vi "infoStepMini.vi"(8 "error in (no error)":errorcluster, 10 "StepId":i32, 11 "Array":T1[](array[typedef])) -> (0 "error out":errorcluster, 3 "Info Test":string)   [LabVIEW 2019]
doc: "Riassume le informazioni principali degli step in un formato più leggibile e ridotto"
uses:
  ByteQXAPIBase/TypeDef/Step.ctl
  ByteQXAPIBase/TypeDef/Asset.ctl
  ByteQXAPIBase/ByteQXAPIBase.lvclass
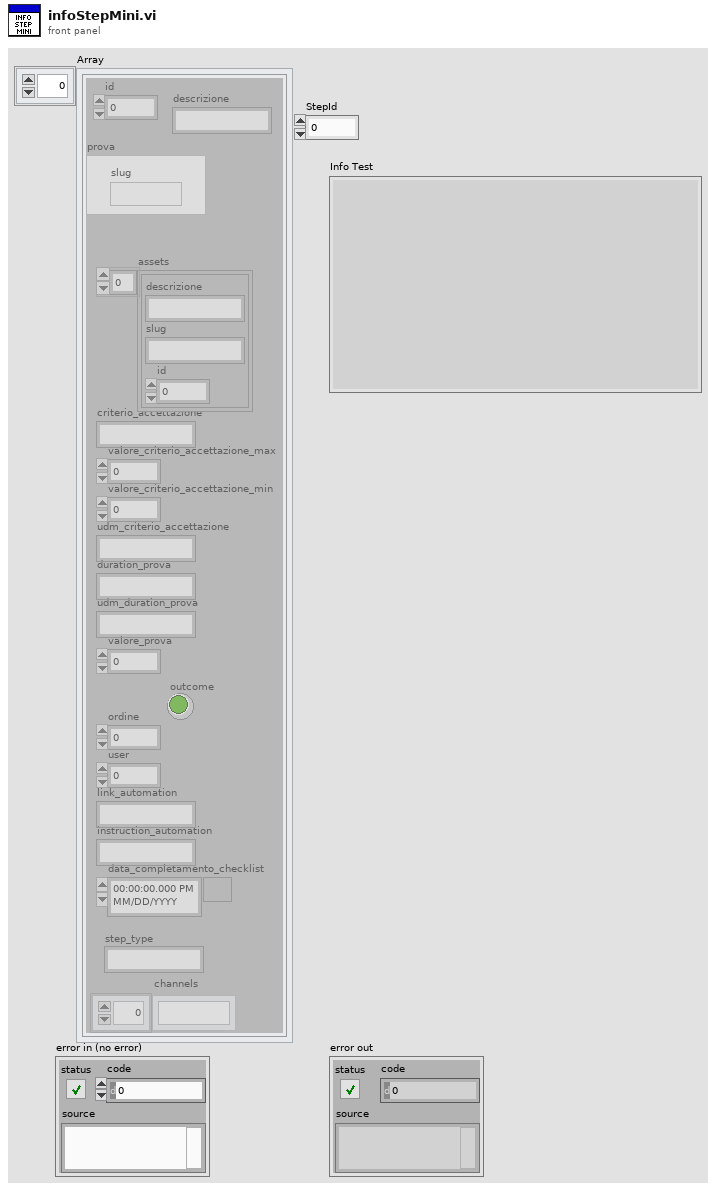
[diagram p1: front panel]
types:
  T1 = typedef "ByteQXWebAPI.lvlib/ByteQXAPIBase.lvclass/Step.ctl" = cluster{"id":i32, "descrizione":string, "prova":cluster{"slug":string}, "assets":T2[], "criterio_accettazione":string, "valore_criterio_accettazione_max":dbl, "valore_criterio_accettazione_min":dbl, "udm_criterio_accettazione":string, "duration_prova":string, "udm_duration_prova":string, "valore_prova":dbl, "ordine":i32, "user":i32, "link_automation":string, "instruction_automation":string, "data_completamento_checklist":timestamp, "outcome":bool, "step_type":string, "channels":string[]}
  T2 = typedef "ByteQXWebAPI.lvlib/ByteQXAPIBase.lvclass/Asset.ctl" = cluster{"descrizione":string, "slug":string, "id":i32}
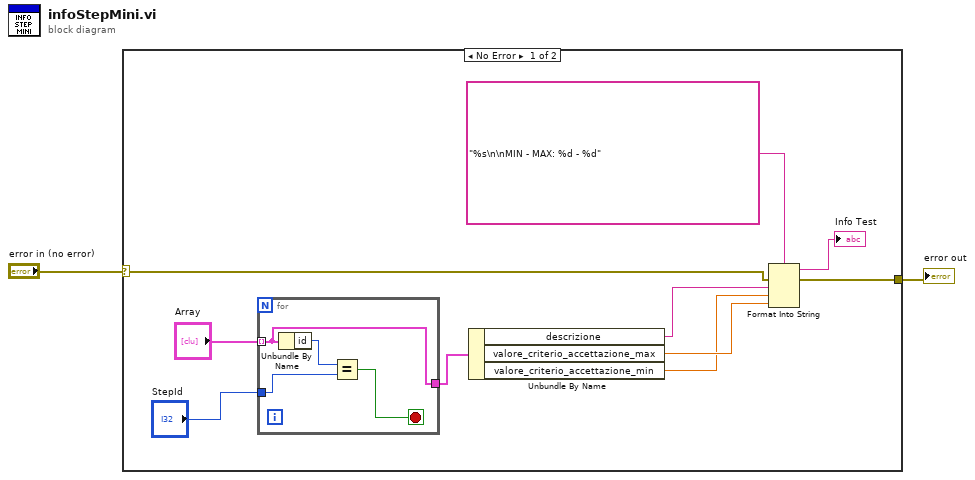
[diagram p0: block diagram]
diagram:
  n1 = case shown="No Error" "error in (no error)" {
    selector: "error in (no error)" -> [w9 w17]
    tunnel: [w8 w17] -> w1
    frame No Error {
      n2 = for {
        tunnel: "Array" -> [w13] mode=indexing
        tunnel: "StepId" -> [w16]
        tunnel: [w13] -> w3
        stop <- w14 stop-if-true
        n3 = Unbundle By Name(w13) -> ("id"=w15:i32)
        n4 = Equal?(x=w15, y=w16) -> (x = y?=w14:bool)
      }
      n5 = Unbundle By Name(w3) -> ("descrizione"=w10:string, "valore_criterio_accettazione_max"=w7:dbl, "valore_criterio_accettazione_min"=w6:dbl)
      n6 = Format Into String(format string="%s\n\nMIN - MAX: %d - %d", error in=w9, w10, w6, w7) -> (resulting string=→"Info Test":string, error out=w8:errorcluster)  [unwired: 1 in]
    }
    frame Error {
    }
  }
  "error out" <- w1
